vi "Read Holding Registers.vi"(8 "error in (no error)":errorcluster, 9 "number of holding registers":u16, 10 "starting address":u16, 11 "Modbus slave in":refnum<class "Modbus Slave.lvclass">) -> (0 "error out":errorcluster, 2 "register values":u16[](array[numeric]), 3 "Modbus slave out":refnum<class "Modbus Slave.lvclass">)   [LabVIEW 2021, in "Modbus Slave.lvclass"]
doc: "Reads values of contiguous holding registers."
uses:
  Modbus Slave.lvclass
  Modbus Slave.lvclass/Modbus Slave.ctl
  Data Model/Device Data Model.lvclass
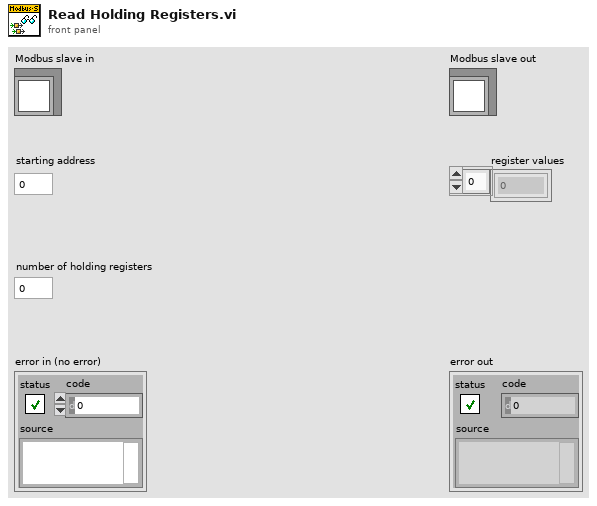
[diagram p1: front panel]
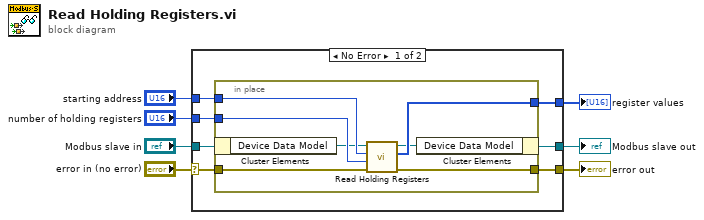
[diagram p0: block diagram]
diagram:
  n1 = case shown="No Error" "error in (no error)" {
    selector: "error in (no error)" -> [w8 w22]
    tunnel: [w14 w22] -> w7
    tunnel: [w13 w23] -> w6
    tunnel: [w12 _] -> w5
    tunnel: "Modbus slave in" -> [w11 w23]
    tunnel: "starting address" -> [w10 _]
    tunnel: "number of holding registers" -> [w9 _]
    frame No Error {
      n2 = in-place {
        in-place-border: [w21] -> w12
        in-place-border: w9 -> [w20]
        in-place-border: w10 -> [w19]
        in-place-border: [w18] -> w14
        in-place-border: w8 -> [w17]
        n3 = in-place-cluster #1(w11) -> ("Device Data Model"=w15:refnum<class "Device Data Model.lvclass">)
        n4 = call-dynamic "Read Holding Registers.vi"("error in"=w17, "number of registers"=w20, "starting address"=w19, "device data model in"=w15) -> ("error out"=w18:errorcluster, "data"=w21:u16[], "device data model out"=w16:refnum<class "Device Data Model.lvclass">)  [unwired: 5 in]
        n5 = in-place-cluster #1("Device Data Model"=w16) -> (w13:refnum<class "Modbus Slave.lvclass">)
      }
    }
    frame Error {
    }
  }
  "error out" <- w7
  "Modbus slave out" <- w6
  "register values" <- w5
